vi "finishUp.vi"(8 "error in (no error)":errorcluster, 11 "ImageStreamViewer in":refnum<class "ImageStreamViewer.lvclass">) -> (0 "error out":errorcluster, 3 "ImageStreamViewer out":refnum<class "ImageStreamViewer.lvclass">)   [LabVIEW 2011, in "Views.lvlib" / "Camera.lvlib" / "ImageStreamViewer.lvclass"]
uses:
  ImageStreamViewer.lvclass
  ImageStreamViewer.lvclass/ImageStreamViewer.ctl
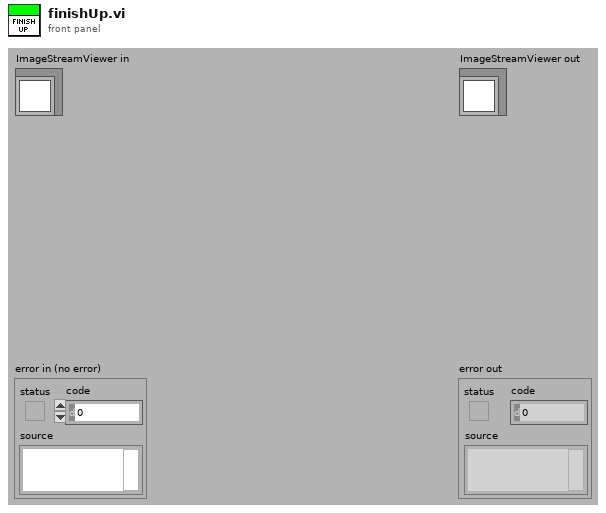
[diagram p1: front panel]
types:
  T1 = typedef "IMAQ Image.ctl" = refnum<image>
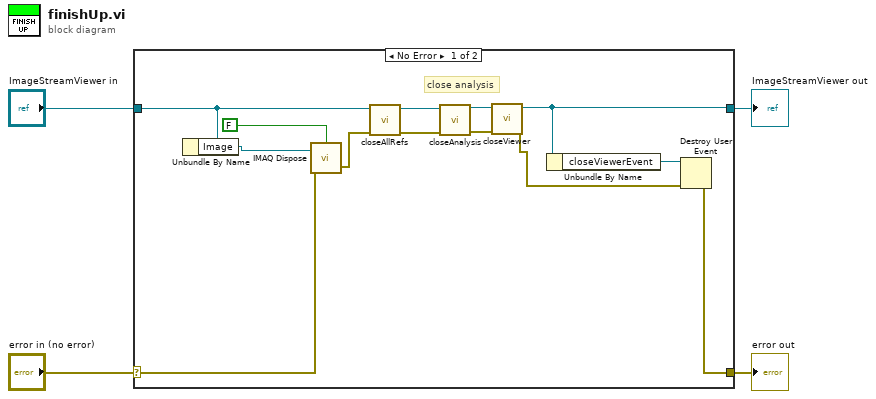
[diagram p0: block diagram]
diagram:
  n1 = case shown="No Error" "error in (no error)" {
    selector: "error in (no error)" -> [w16 w19]
    tunnel: [w5 w19] -> w3
    tunnel: [w8 w18] -> w1
    tunnel: "ImageStreamViewer in" -> [w14 w18]
    frame No Error {
      # "close analysis"
      n2 = Unbundle By Name(w14) -> ("Image"=w17:T1)
      n3 = call "IMAQ Dispose"("All Images? (No)"=FALSE, "Image"=w17, "error in (no error)"=w16) -> ("error out"=w13:errorcluster)  [unwired: 3 in]
      n4 = call "closeAllRefs.vi"("error in (no error)"=w13, "ImageStreamViewer in"=w14) -> ("error out"=w11:errorcluster, "ImageStreamViewer out"=w12:refnum<class "ImageStreamViewer.lvclass">)  [unwired: 8 in]
      n5 = call "closeAnalysis.vi"("error in (no error)"=w11, "ImageStreamViewer in"=w12) -> ("error out"=w9:errorcluster, "ImageStreamViewer out"=w10:refnum<class "ImageStreamViewer.lvclass">)  [unwired: 8 in]
      n6 = call "closeViewer.vi"("error in (no error)"=w9, "ImageStreamViewer in"=w10) -> ("error out"=w6:errorcluster, "ImageStreamViewer out"=w8:refnum<class "ImageStreamViewer.lvclass">)  [unwired: 8 in]
      n7 = Unbundle By Name(w8) -> ("closeViewerEvent"=w7:refnum<user-event>)
      n8 = Destroy User Event(user event=w7, error in=w6) -> (error out=w5:errorcluster)
    }
    frame Error {
    }
  }
  "error out" <- w3
  "ImageStreamViewer out" <- w1
